vi "TPFLSHdll_d.vi"(5 "dll_path_in":path, 8 "error in (no error)":errorcluster, 9 "Component Molar Fractions":dbl[](array[numeric])=[1.0, 0.0, 0.0, 0.0, 0.0, 0.0, 0.0, 0.0, 0.0, 0.0, 0.0, 0.0, 0.0, 0.0, 0.0, 0.0, 0.0, 0.0, 0.0, 0.0], 10 "p":dbl, 11 "Temp (deg c)":dbl=30.0) -> (0 "error out":errorcluster, 3 "TPDATAOUT":dbl[](array[numeric]), 4 "dll_path_out":path)   [LabVIEW 2017]
doc: "Please feel free to contact me if you have any questions .\nMy mail:ken_pop@tom.com yan.ding@jci.com"
panel:
  out "x":dbl[](array[numeric])
  out "d":dbl
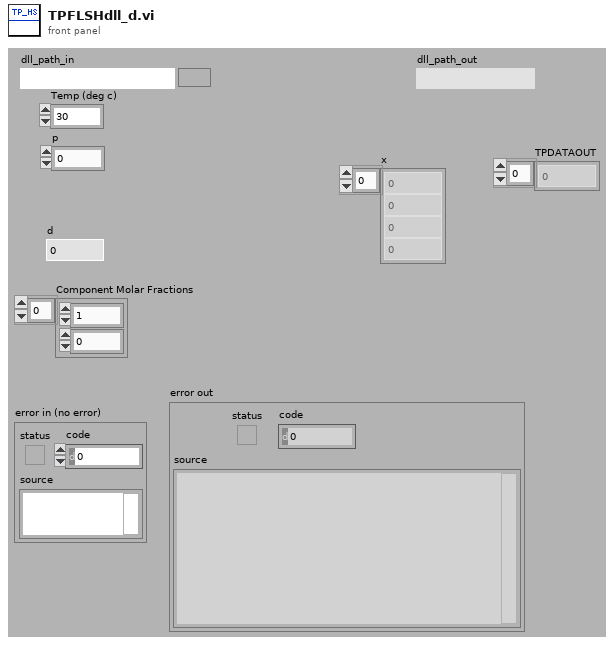
[diagram p1: front panel]
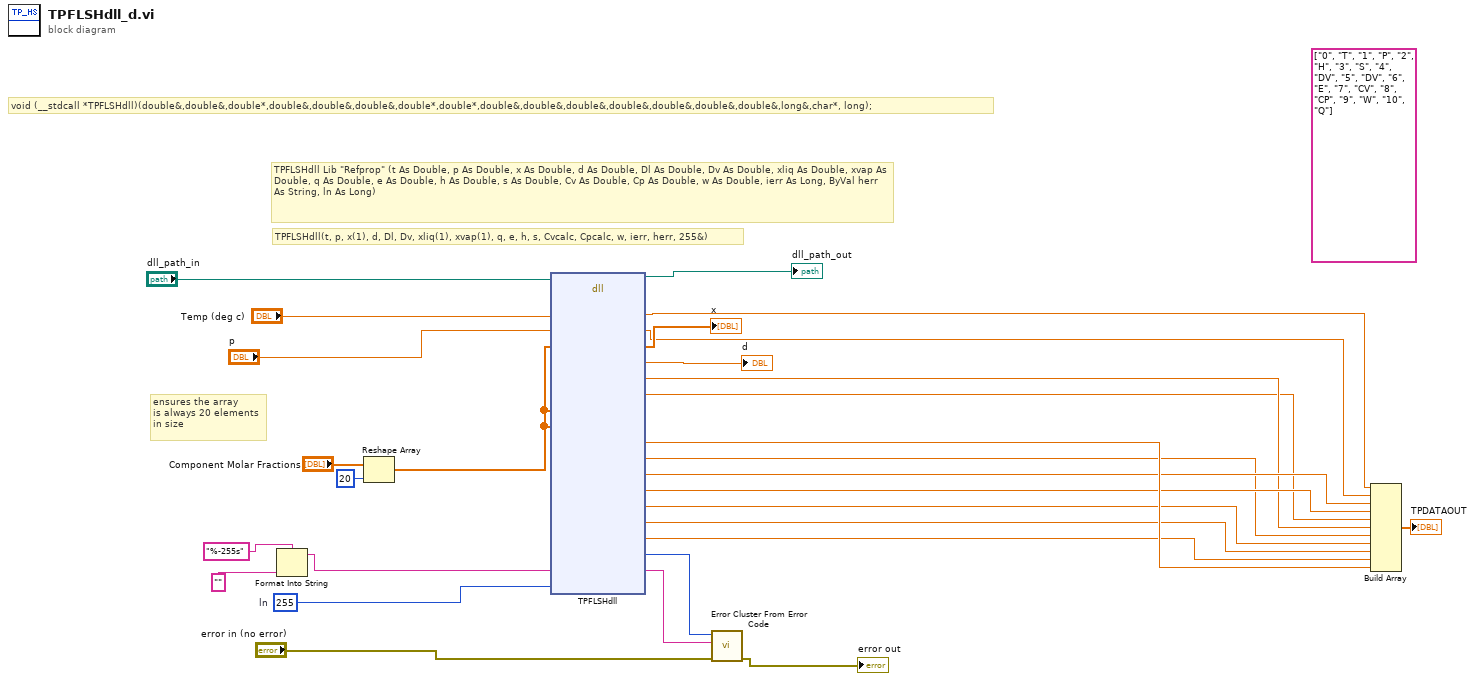
[diagram p0: block diagram]
diagram:
  (unwired) string[][] [["0", "T"], ["1", "P"], ["2", "H"], ["3", "S"], ["4", "DV"], ["5", "DV"], ["6", "E"], ["7", "CV"], ["8", "CP"], ["9", "W"], ["10", "Q"]] ("数组")
  w21 = 255  # ln
  # "void (__stdcall *TPFLSHdll)(double&,double&,double*,double&,double&,double&,double*,double*,double&,double&,double&,double&,double&,double&,double&,long&,char*, long);"
  # "TPFLSHdll Lib \"Refprop\" (t As Double, p As Double, x As Double, d As Double, Dl As Double, Dv As Double, xliq As Double, xvap As Double, q As Double, e As Double, h As Double, s As Double, Cv As Double, Cp As Double, w As Double, ierr As Long, ByVal herr As String, ln As Long)"
  # "TPFLSHdll(t, p, x(1), d, Dl, Dv, xliq(1), xvap(1), q, e, h, s, Cvcalc, Cpcalc, w, ierr, herr, 255&)"
  # "ensures the array\nis always 20 elements\nin size"
  n1 = Format Into String(format string="%-255s", "") -> (resulting string=w20:string)  [unwired: 2 in, 1 out]
  n2 = Reshape Array("Component Molar Fractions", 20 ("dimension size")) -> (w17:dbl[])
  n3 = dll-call lib="refprop.DLL" fn="TPFLSHdll"(path in="dll_path_in", "t"="Temp (deg c)", "p"="p", "x"=w17, "xliq"=w17, "xvap"=w17, "herr"=w20, "ln"=w21) -> (path out=→"dll_path_out":path, "t"=w12:dbl, "p"=w14:dbl, "x"=→"x":dbl[], "d"=→"d":dbl, "Dl"=w9:dbl, "Dv"=w4:dbl, "q"=w13:dbl, "e"=w8:dbl, "h"=w11:dbl, "s"=w10:dbl, "cv"=w7:dbl, "cp"=w6:dbl, "w"=w5:dbl, "ierr"=w22:i32, "herr"=w23:string)  [unwired: 17 in, 1 out]
  n4 = call <vilib>:"Error Cluster From Error Code.vi"("error in (no error)"="error in (no error)", "error message (\"\")"=w23, "error code (0)"=w22) -> ("error out"=→"error out":errorcluster)  [unwired: 6 in]
  n5 = Build Array(w12, w14, w11, w10, w4, w9, w8, w7, w6, w5, w13) -> (→"TPDATAOUT":dbl[])
